vi "sbRIO Status.vi"(8 "error in (no error)":errorcluster, 11 "Refnum in":T1) -> (0 "error out":errorcluster, 2 "Subsystem Status":T2, 3 "Refnum out":T1)   [LabVIEW 2014]
uses:
  Subsystem Status.ctl
  Subsystem Status Severity.ctl
  Subsystem Status Message.ctl
  FPGA Typedef.ctl
  <vilib>/Utility/error.llb/Error Cluster From Error Code.vi
  <vilib>/rvi/errors/niLvFpgaAdjustHostInterfaceError.vi
  <vilib>/rvi/interface/nirviReadWriteControl/nirviReadWriteControl.xnode
  FPGA Bitfiles/Latest.lvbitx
  NiFpgaLv.dll
panel:
  in  "Low Battery Thres.":fxp<+/-,25,6>=12.200000762939453
  in  "sbRIO Overheat Thres.":fxp<+/-,33,17>=75.0
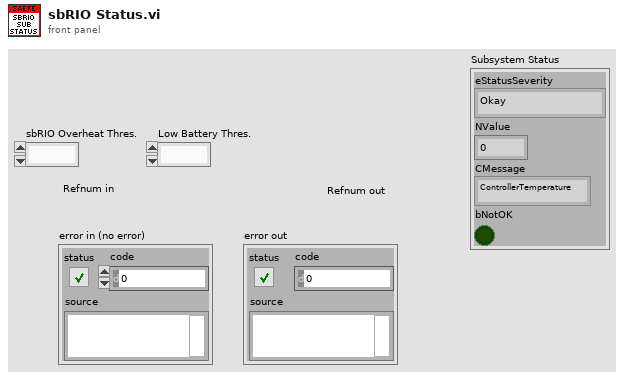
[diagram p1: front panel]
types:
  T1 = typedef "FPGA Typedef.ctl" = refnum<k20>
  T2 = typedef "Subsystem Status.ctl" = cluster{"eStatusSeverity":T3, "NValue":sgl, "CMessage":T4, "bNotOK":bool}
  T3 = typedef "Subsystem Status Severity.ctl" = enum16{"Okay", "Short Warning", "Long Warning", "Return to Pits", "Error", "Danger"}
  T4 = typedef "Subsystem Status Message.ctl" = enum16{"ControllerTemperature", "MotorTemperature", "BatteryTemperature", "BatteryLowVoltage", "LVBattery", "sbRIOTemperature", "Precharge", "BSPD", "IMD", "RemoteReturnToPits", "EStopInterrupted", "NoCellComms", "MCOverSpeed", "MCOverCurrent", "MCOverVoltage", "MCInverterOverTemp", "MCDirectionCommand", "MCInverterTimeout", "MCDesatFault", "MCHWOverCurrent", "MCUnderVoltage", "MCCommandMessageLost", "MotorOverTemp", "MCModAOverTemp", "MCModBOverTemp", "MCModCOverTemp", "MCPCBOverTemp", "MCGateDrv1OverTemp", "MCDateDrv2OverTemp", "MCCurrentSensorFault", "MCResolverNotConnected", "ShutdownLatchTripped", "UnknownBMS", "RemoteEmergency"}
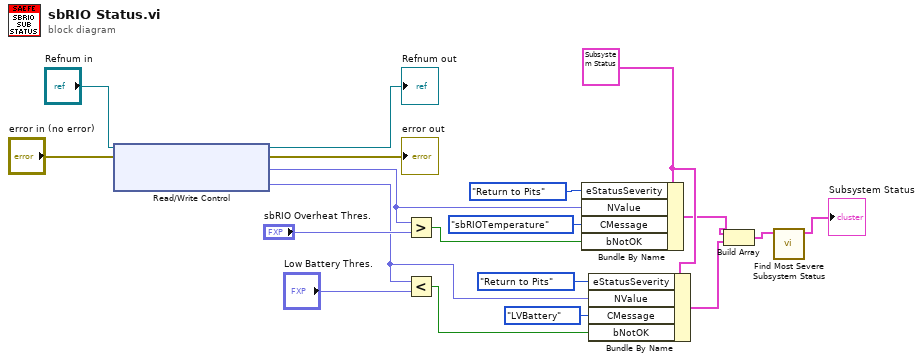
[diagram p0: block diagram]
diagram:
  w9 = T2 {"eStatusSeverity"=enum."Okay", "NValue"=0.0, "CMessage"=enum."ControllerTemperature", "bNotOK"=FALSE} ("Subystem Status")
  n1 = xnode "Read/Write Control"("FPGA VI Reference In"="Refnum in", "error in"="error in (no error)") -> ("FPGA VI Reference Out"=→"Refnum out":T1, "error out"=→"error out":errorcluster, "TSBRIO"=w13:fxp<+,19,8>, "VsbRIOSupply"=w8:fxp<+/-,25,6>)
  n2 = Greater?(x=w13, y="sbRIO Overheat Thres.") -> (0:w10:bool)
  n3 = Less?(x=w8, y="Low Battery Thres.") -> (x < y?=w5:bool)
  n4 = Bundle By Name(cluster=w9, "eStatusSeverity"=Subsystem_Status_Severity."Return to Pits" ("Status Severity"), "NValue"=w13, "CMessage"=Subsystem_Status_Message."sbRIOTemperature" ("Message"), "bNotOK"=w10) -> (w4:T2)
  n5 = Bundle By Name(cluster=w9, "eStatusSeverity"=Subsystem_Status_Severity."Return to Pits" ("Status Severity"), "NValue"=w8, "CMessage"=Subsystem_Status_Message."LVBattery" ("Message"), "bNotOK"=w5) -> (w3:T2)
  n6 = Build Array(w4, w3) -> (w2:T2[])
  n7 = call "Find Most Severe Subsystem Status.vi"("Array"=w2) -> ("Subystem Status"=→"Subsystem Status":T2)  [unwired: 10 in]
